vi "Memory.Pointer.Write.Unsafe.1D.I64.vi"(8 "error in (no error)":errorcluster, 9 "count":u64 format="%d elements", 10 "buffer in":i64[](array[numeric]), 11 "pointer in":refnum<class "Memory.Pointer.lvclass">) -> (0 "error out":errorcluster, 2 "buffer out":i64[](array[numeric]), 3 "pointer out":refnum<class "Memory.Pointer.lvclass">)   [LabVIEW 2016, in "Memory Manager.lvlib" / "Memory.Pointer.lvclass"]
doc: "Writes <b>count</b> elements from the provided <b>buffer</b> to the address specified by <b>pointer</b>.\n\n<b>Note:</b> This VI is <b>unsafe</b>.\n\nUnsafe means that it does not evaluate the size parameter of <b>pointer</b> to ensure that is inbounds of allocated memory before peforming a memory read/write. Reading/writing more data to a pointer than it has allocated can corrupt or crash LabVIEW. Only use this VI in scenarios where the <b>pointer</b> has been validated to be allocated to a correct size before calling this VI."
uses:
  Memory.Pointer.lvclass
  Memory.Pointer.lvclass/Memory.Pointer.ctl
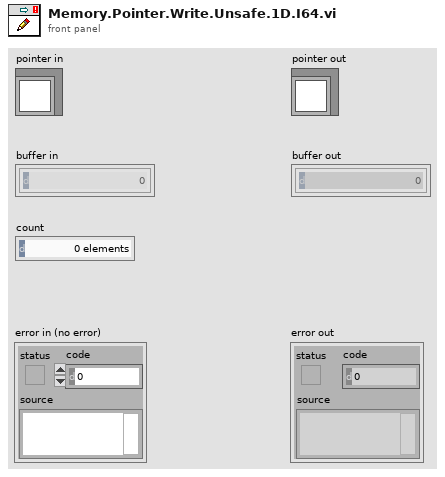
[diagram p1: front panel]
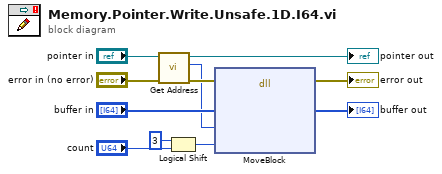
[diagram p0: block diagram]
diagram:
  n1 = call "Get Address.vi"("error in (no error)"="error in (no error)", "Pointer in"="pointer in") -> ("error out"=w10:errorcluster, "address"=w1:u64, "Pointer out"=→"pointer out":refnum<class "Memory.Pointer.lvclass">)  [unwired: 7 in]
  n2 = Logical Shift(y=i16 3, x="count") -> (x << y=w3:u64)
  n3 = dll-call lib="LabVIEW" fn="MoveBlock"(error in=w10, "src"="buffer in", "dst"=w1, "size"=w3) -> (error out=→"error out":errorcluster, "src"=→"buffer out":i64[])  [unwired: 5 in, 1 out]
